vi "Create.vi"(7 "VolatusAPI":refnum<class "VolatusAPI.lvclass">, 8 "error in (no error)":errorcluster, 10 "Config Element":refnum<class "Config Element.lvclass">) -> (0 "error out":errorcluster, 3 "PV Calc out":refnum<class "PV Calc.lvclass">)   [LabVIEW 2020, in "VolatusControl.lvlib" / "PV Calc.lvclass"]
uses:
  PV Calc.lvclass
  PV Calc.lvclass/PV Calc.ctl
  lv-cdm/CDM-Config/Config Element/Config Element.lvclass
  Calc Type.ctl
  Volatus/VolatusAPI/VolatusAPI.lvclass
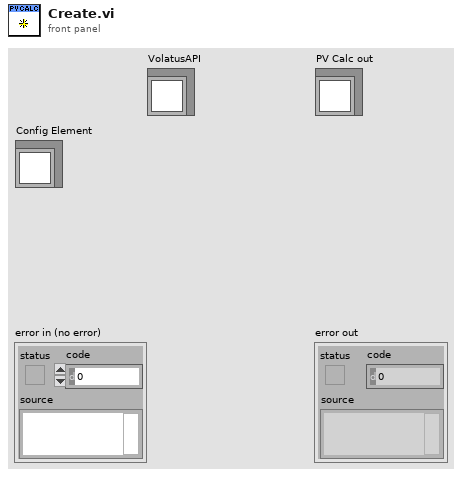
[diagram p1: front panel]
types:
  T1 = typedef "VolatusControl.lvlib/PV Calc.lvclass/Calc Type.ctl" = enum16{"Average", "Median", "Min", "Max"}
  T2 = typedef "CDM-Config.lvlib/Value Type.ctl" = enum16{"String", "Number", "Bool", "Object", "Array"}
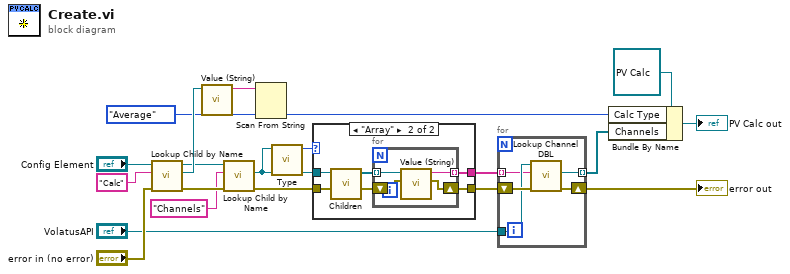
[diagram p0: block diagram]
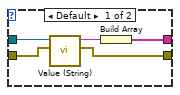
[diagram p2: hidden frame]
diagram:
  n1 = call "Lookup Child by Name.vi"("error in (no error)"="error in (no error)", "Name"="Calc", "Config Element in"="Config Element") -> ("error out"=w13:errorcluster, "Child"=w17:refnum<class "Config Element.lvclass">, "Config Element out"=w14:refnum<class "Config Element.lvclass">)  [unwired: 5 in, 1 out]
  n2 = call "Value (String).vi"("Config Element in"=w17) -> ("String Value"=w16:string)  [unwired: 9 in, 1 out]
  n3 = call "Lookup Child by Name.vi"("error in (no error)"=w13, "Name"="Channels", "Config Element in"=w14) -> ("error out"=w10:errorcluster, "Child"=w11:refnum<class "Config Element.lvclass">)  [unwired: 5 in, 2 out]
  n4 = Scan From String(input string=w16, default 1=Calc_Type."Average" ("Calc Type")) -> (output 1=w8:T1)  [unwired: 3 in, 3 out]
  n5 = call "Type.vi"("Config Element in"=w11) -> ("Value Type"=w12:T2)  [unwired: 9 in, 1 out]
  n6 = case shown="\"Array\"" w12 {
    tunnel: w11 -> [w25 w30]
    tunnel: w10 -> [w24 w27]
    tunnel: [w22 w28] -> w6
    tunnel: [w21 w26] -> w5
    frame Default {
      n7 = call "Value (String).vi"("error in (no error)"=w24, "Config Element in"=w25) -> ("error out"=w21:errorcluster, "String Value"=w23:string)  [unwired: 8 in]
      n8 = Build Array(w23) -> (w22:string[])
    }
    frame "Array" {
      n9 = call "Children.vi"("Config Element in"=w30) -> ("Elements"=w29:refnum<class "Config Element.lvclass">[])  [unwired: 9 in, 1 out]
      n10 = for {
        tunnel: w29 -> [w34] mode=indexing
        tunnel: [w33] -> w28 mode=indexing
        shift-right: [w31] -> w26
        shift-left: w27 -> [w32]
        n11 = call "Value (String).vi"("error in (no error)"=w32, "Config Element in"=w34) -> ("error out"=w31:errorcluster, "String Value"=w33:string)  [unwired: 8 in]
      }
    }
  }
  n12 = for {
    tunnel: "VolatusAPI" -> [w38]
    tunnel: w6 -> [w37] mode=indexing
    shift-right: [w36] -> w3
    shift-left: w5 -> [w39]
    tunnel: [w35] -> w4 mode=indexing
    n13 = call "Lookup Channel DBL.vi"("error in (no error)"=w39, "Name"=w37, "VolatusAPI in"=w38) -> ("error out"=w36:errorcluster, "Channel DBL"=w35:refnum<class "Channel DBL.lvclass">)  [unwired: 6 in, 1 out]
  }
  "error out" <- w3
  n14 = Bundle By Name(cluster=refnum<class "PV Calc.lvclass"> refnum ("PV Calc in"), "Calc Type"=w8, "Channels"=w4) -> (→"PV Calc out":refnum<class "PV Calc.lvclass">)
